vi "OpenMono.vi"(0 "Mono Port":refnum<visa-resource-name>) -> (1 "VISA resource name out":refnum<visa-resource-name>, 2 "error out":errorcluster)   [LabVIEW 2009]
uses:
  <vilib>/Instr/_visa.llb/VISA Configure Serial Port (Instr).vi
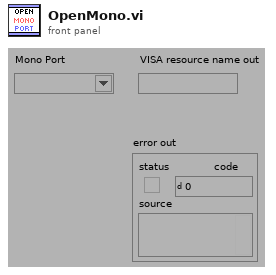
[diagram p1: front panel]
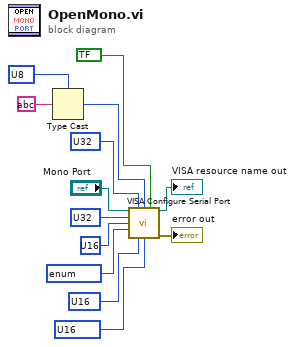
[diagram p0: block diagram]
diagram:
  w3 = u16 ? items=["None", "XON/XOFF", "RTS/CTS", "XON/XOFF & RTS/CTS", "DTR/DSR", "XON/XOFF & DTR/DSR"] ("flow control (0:none)")
  w5 = u16 ? items=["1.0", "1.5", "2.0"] ("stop bits (10: 1 bit)")
  n1 = Type Cast(type=u8 ? ("timeout (10sec)"), x=string ?) -> (*(type *) &x=w9:u8)
  n2 = call-poly "VISA Configure Serial Port"("VISA resource name"="Mono Port", "timeout (10sec)"=u32 ?, "termination char\n(0xA = '\\n' = LF)"=w9, "Enable Termination\nChar (T)"=bool ? ("Enable Termination\nChar (T)"), "baud rate (9600)"=u32 ?, "data bits (8)"=u16 ?, "parity (0:none)"=enum16{"None", "Odd", "Even", "Mark", "Space"} ?, "stop bits (10: 1 bit)"=w5, "flow control (0:none)"=w3) -> ("VISA resource name out"=→"VISA resource name out":refnum<visa-resource-name>, "error out"=→"error out":errorcluster)  [unwired: 5 in]
